vi "Configure Digital Inputs.vi"(0 "VISA resource name":refnum<visa-resource-name>, 1 "Input Connector Select (0: dioC0)":i32(ring) items=["dioC0", "dioC1"], 2 "Input Num Bits (0)":i32, 3 "Input Term (T: Enable)":i32(ring) items=["dinHiZ", "dinLoZ"], 5 "Deemphasis (0: dioNoDeem)":i32(ring) items=["dioNoDeem", "dioCD501dB0", "dioCD501dB10", "dioJ17dB0", "dioJ17dB20"], 7 "Input Block DC (T: Enable)":bool=TRUE, 9 "Input Carrier EQ (T: Enable)":bool=TRUE, 11 "error in (no error)":errorcluster, 12 "Input Dual Connector (T: Enable)":bool=TRUE, 13 "Input Source (0: dioXlR)":i32(ring) items=["dioXlR", "diBNC", "diOptical", "diGenMin", "diNone"]) -> (4 "VISA resource name out":refnum<visa-resource-name>, 15 "error out":errorcluster)   [LabVIEW 2014, in "Stanford Research SR1.lvlib"]
doc: "Configures the basic attributes for the Digital inputs."
uses:
  Stanford Research SR1.lvlib
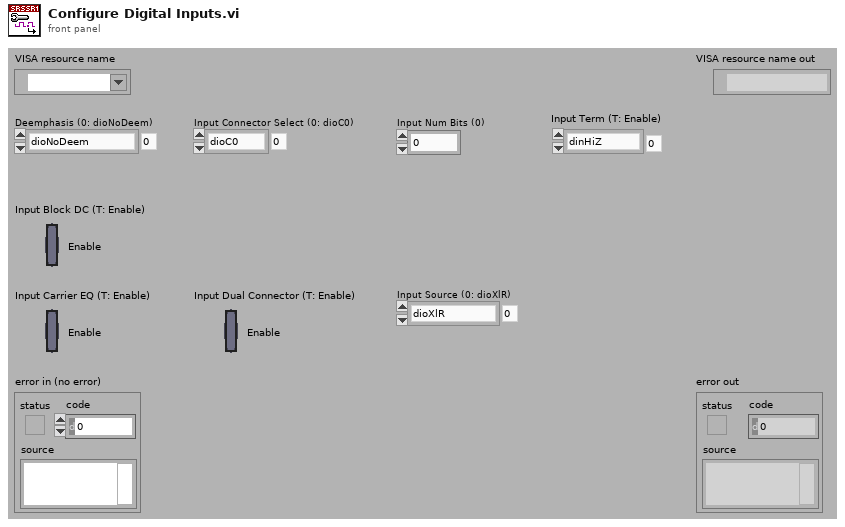
[diagram p1: front panel]
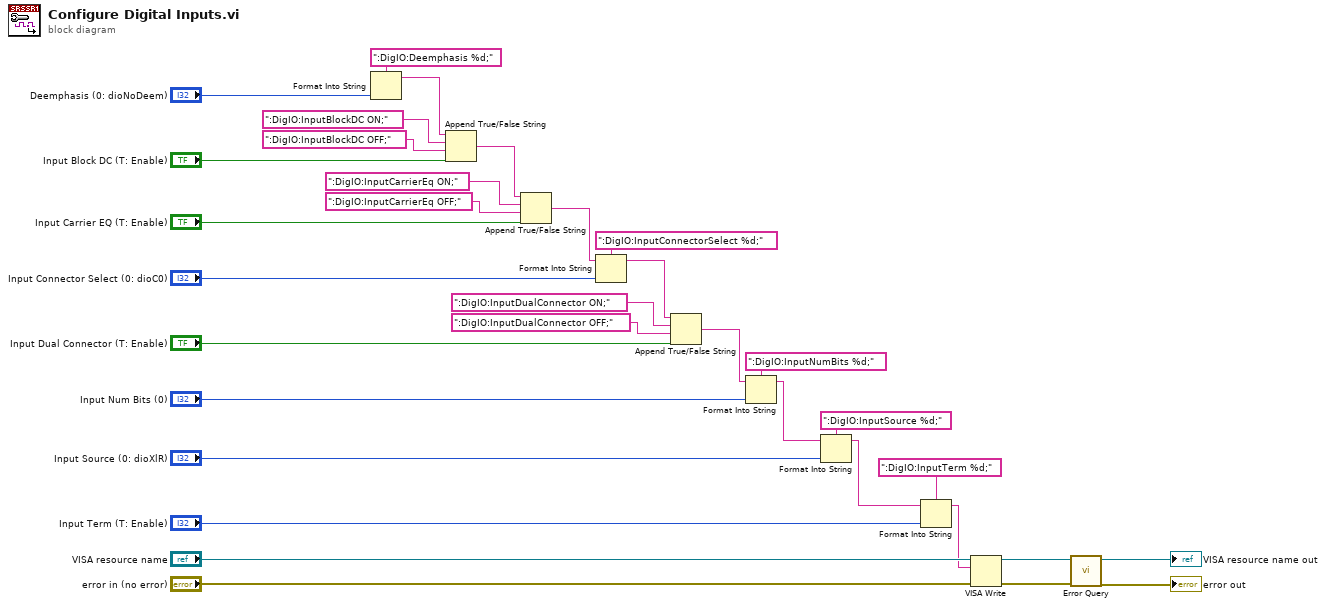
[diagram p0: block diagram]
diagram:
  n1 = Format Into String(format string=":DigIO:Deemphasis %d;", "Deemphasis (0: dioNoDeem)") -> (resulting string=w31:string)  [unwired: 2 in, 1 out]
  n2 = Append True/False String(1:"Input Block DC (T: Enable)", 2:":DigIO:InputBlockDC OFF;", 3:":DigIO:InputBlockDC ON;", 4:w31) -> (0:w27:string)
  n3 = Append True/False String(1:"Input Carrier EQ (T: Enable)", 2:":DigIO:InputCarrierEq OFF;", 3:":DigIO:InputCarrierEq ON;", 4:w27) -> (0:w23:string)
  n4 = Format Into String(format string=":DigIO:InputConnectorSelect %d;", initial string=w23, "Input Connector Select (0: dioC0)") -> (resulting string=w20:string)  [unwired: 1 in, 1 out]
  n5 = Append True/False String(1:"Input Dual Connector (T: Enable)", 2:":DigIO:InputDualConnector OFF;", 3:":DigIO:InputDualConnector ON;", 4:w20) -> (0:w16:string)
  n6 = Format Into String(format string=":DigIO:InputNumBits %d;", initial string=w16, "Input Num Bits (0)") -> (resulting string=w13:string)  [unwired: 1 in, 1 out]
  n7 = Format Into String(format string=":DigIO:InputSource %d;", initial string=w13, "Input Source (0: dioXlR)") -> (resulting string=w4:string)  [unwired: 1 in, 1 out]
  n8 = Format Into String(format string=":DigIO:InputTerm %d;", initial string=w4, "Input Term (T: Enable)") -> (resulting string=w1:string)  [unwired: 1 in, 1 out]
  n9 = VISA Write(VISA resource name="VISA resource name", write buffer=w1, error in (no error)="error in (no error)") -> (VISA resource name out=w8:refnum<visa-resource-name>, error out=w7:errorcluster)  [unwired: 1 out]
  n10 = call "Error Query.vi"("error in (no error)"=w7, "VISA resource name"=w8) -> ("error out"=→"error out":errorcluster, "VISA resource name out"=→"VISA resource name out":refnum<visa-resource-name>)  [unwired: 6 in, 2 out]
